vi "libssh2_channel_flush_ex.vi"(8 "error in (no error)":errorcluster, 10 "streamid":i32, 11 "channel":T1) -> (0 "error out":errorcluster)   [LabVIEW 2013, in "libssh2.lvlib"]
doc: "Flush the read buffer for a channel."
uses:
  libssh2.lvlib
  Channel Refnum.ctl
  Not A Channel.vi
  <vilib>/Utility/error.llb/Error Cluster From Error Code.vi
  Global Settings.vi
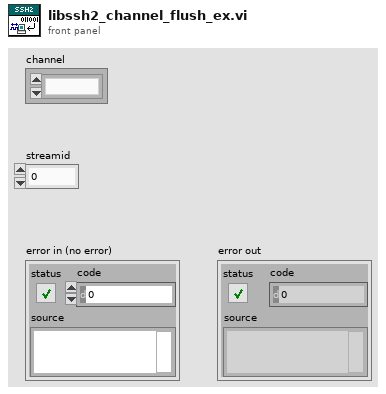
[diagram p1: front panel]
types:
  T1 = typedef "libssh2.lvlib/Channel Refnum.ctl" = refnum<k1>
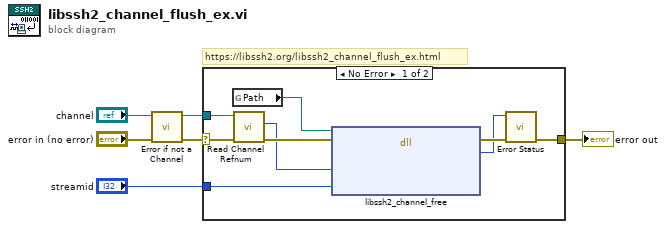
[diagram p0: block diagram]
diagram:
  # "https://libssh2.org/libssh2_channel_flush_ex.html"
  n1 = call "Error if not a Channel.vi"("error in (no error)"="error in (no error)", "channel"="channel") -> ("error out"=w3:errorcluster, "channel out"=w1:T1)  [unwired: 8 in]
  n2 = case shown="No Error" w3 {
    selector: w3 -> [w14 w16]
    tunnel: [w13 w16] -> w6
    tunnel: "streamid" -> [w15 _]
    tunnel: w1 -> [w12 _]
    frame No Error {
      n3 = global read "Global Settings.vi" "Path"() -> (w8:path)
      n4 = call "Read Channel Refnum.vi"("error in (no error)"=w14, "channel"=w12) -> ("error out"=w10:errorcluster, "LIBSSH2_CHANNEL*"=w9:u64)  [unwired: 8 in]
      n5 = dll-call lib="?" fn="libssh2_channel_free"(path in=w8, error in=w10, "channel"=w9, "streamid"=w15) -> (error out=w11:errorcluster, "return value"=w7:i32)  [unwired: 3 in, 1 out]
      n6 = call "Error Status.vi"("error in (no error)"=w11, "return value"=w7) -> ("error out"=w13:errorcluster)  [unwired: 8 in, 1 out]
    }
    frame Error {
    }
  }
  "error out" <- w6
